vi "Get Unitless Values.vi"(8 "error in (no error)":errorcluster, 11 "Analyze Results Fluence and Energy in":refnum<class "Analyze Results Fluence and Energy.lvclass">) -> (0 "error out":errorcluster, 2 "UnitLess Values":T1[](array[typedef]), 3 "Analyze Results Fluence and Energy out":refnum<class "Analyze Results Fluence and Energy.lvclass">)   [LabVIEW 2020, in "Analyze Results Fluence and Energy.lvclass"]
uses:
  Analyze Results Fluence and Energy.lvclass
  Results Base/UnitLessValue.ctl
  Results Fluence/Analyze Results Fluence.lvclass
  Results Base/Analyze Results Base.lvclass
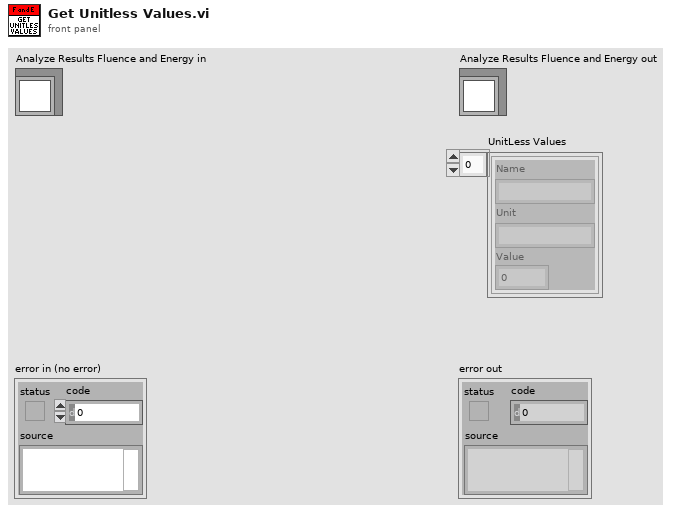
[diagram p1: front panel]
types:
  T1 = typedef "Analyze Results Base.lvclass/UnitLessValue.ctl" = cluster{"Name":string, "Unit":string, "Value":dbl}
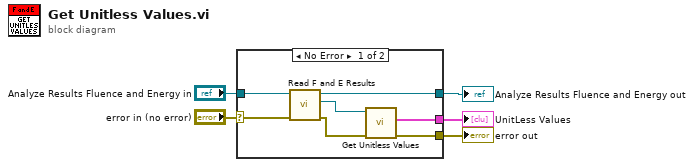
[diagram p0: block diagram]
diagram:
  n1 = case shown="No Error" "error in (no error)" {
    selector: "error in (no error)" -> [w10 w13]
    tunnel: "Analyze Results Fluence and Energy in" -> [w11 w14]
    tunnel: [w12 w14] -> w4
    tunnel: [w7 w13] -> w2
    tunnel: [w6 _] -> w1
    frame No Error {
      n2 = call "Read F and E Results.vi"("error in (no error)"=w10, "Analyze Results Fluence and Energy in"=w11) -> ("error out"=w8:errorcluster, "Fluence"=w9:refnum<class "Analyze Results Fluence.lvclass">, "Analyze Results Fluence and Energy out"=w12:refnum<class "Analyze Results Fluence and Energy.lvclass">)  [unwired: 6 in, 1 out]
      n3 = call-dynamic "Get Unitless Values.vi"("error in (no error)"=w8, "Analyze Results Fluence in"=w9) -> ("error out"=w7:errorcluster, "UnitLess Values"=w6:T1[])  [unwired: 7 in, 1 out]
    }
    frame Error {
    }
  }
  "error out" <- w2
  "Analyze Results Fluence and Energy out" <- w4
  "UnitLess Values" <- w1
